vi "AlliGator Save IRFs & Fit Data (Map) HDF5 File v0.6.vi"(0 "File Path":path, 5 "IRFs & Fit Data Map v3":T12 {"Fit Options: Decay Preprocessing Parameters"."# Folds" min=1}, 7 "Decay Fit Options & Parameters v3":T1={"SYNC Period"=0.0, "Fit Options"={"Show Fit Residuals"=FALSE, "Fit Model"=enum."1-Exponential", "Residual Type"=enum."Standard", "Max Decay Percentile"=0.0, "Min Decay Percentile"=0.0, "Show Full Decay"=FALSE, "Weights"=enum."Unweighted", "Fitting Method"=enum."Least Square", "Compute Parameter Uncertainties"=FALSE, "Periodic Boundaries"=FALSE, "Model Calculation"=enum."Simulation", "Period"=0.0, "Termination Criteria"={"Max Iterations"=0, "Max Function Calls"=0, "Max Time"=0.0, "Function Tolerance"=0.0, "Parameter Tolerance"=0.0, "Gradient Tolerance"=0.0, "Min Lambda"=0.0, "Max Lambda"=0.0, "Initial Tick Count"=0}, "Offset Resolution"=0.0, "Use Local IRF"=FALSE, "Fitting Algorithm"=enum."Levenberg-Marquardt", "Show Confidence Interval "=TRUE, "Confidence Level"=95.0}, "Fit Parameter Constraints"=[], "MLE Baseline Offset"=0.0, "MLE Baseline Offset Type"=enum."Absolute"} {"Fit Options"."Confidence Level" min=0.0 max=100.0; "Fit Options"."Offset Resolution" min=0.0; "Fit Options"."Period" min=0.0; "Fit Options"."Min Decay Percentile" min=0.0 max=1.0; "Fit Options"."Max Decay Percentile" min=0.0 max=100.0; "Fit Parameter Constraints"."Max Value" format="%#.3g"; "Fit Parameter Constraints"."Min Value" format="%#.3g"}, 9 "Software + Version":string, 11 "Error In":errorcluster, 12 "[Multiple Decays Fit Parameters SDV]":dbl[][](array[numeric])) -> (4 "File Path out":path, 14 "Time (s)":dbl, 15 "Error Out":errorcluster)   [LabVIEW 2021, in "AlliGator Decay Fit Parameter Map.lvlib"]
doc: "Saves Decay Fit Parameter Map and associated metadata to an HDF5 file."
uses:
  AlliGator Decay Fit Parameter Map.lvlib
  Fits/IRF(X)PSED/Decay Fit Parameters & Derived Quantities List v2.ctl
  Decay Analysis/Decay Preprocessing/AlliGator Decay Preprocessing Parameters.ctl
  Graphs/XY Graph/XY Graph Plot Shift Parameters.ctl
  Graphs/XY Graph/XY Graph Plot Shift Method.ctl
  AlliGator Decay Fit Options & Parameters v3.ctl
  Fits/IRF(X)PSED/Decay Fit Options v3.ctl
  Fits/Decay Convolution/Decay Model.ctl
  Fits/Residual Type.ctl
  Fits/IRF(X)PSED/Fit Weights Type.ctl
  Fits/Non-linear Fitting Method v2.ctl
  Fits/Fit Calculation Method.ctl
  Fits/Non-linear Fitting Algorithm.ctl
  Decay Analysis/Decay Fit/AlliGator Decay Fit Parameter Constraints 2.ctl
  Fits/IRF(X)PSED/Decay Fit Parameters In List.ctl
  Fits/IRF(X)PSED/MLE Baseline Offset Type.ctl
  <vilib>/addons/h5labview2/file/H5Fmode.ctl
  Globals, Variables, Constants/AlliGator Variables List.ctl
  <vilib>/addons/h5labview2/base/lib_path.vi
  <vilib>/addons/h5labview2/base/H5Equery.vi
  <vilib>/addons/h5labview2/dataset/H5Dwrite.llb/H5Dwrite.xnode
  <vilib>/addons/h5labview2/base/hid_t.ctl
  Variant/Variant to Data/Variant to String.vi
  <vilib>/addons/h5labview2/file/H5F.lvlib
  <vilib>/addons/h5labview2/group/H5G.lvlib
  Time/Time.lvlib
  Utilities/Utilities.lvlib
  Strings/Strings.lvlib
  Globals, Variables, Constants/AlliGator Globals, Variables & Constants.lvlib
  Variant/Variant to Data/Variant to Data.lvlib
  Fits/Fits.lvlib
  Graphs/XY Graph/XY Graph Add-Ons.lvlib
  Decay Analysis/Decay Preprocessing/AlliGator Decay Preprocessing.lvlib
  Decay Analysis/Decay Fit/AlliGator Decay Fit.lvlib
  AlliGator IRFs & Fit Data v3.ctl
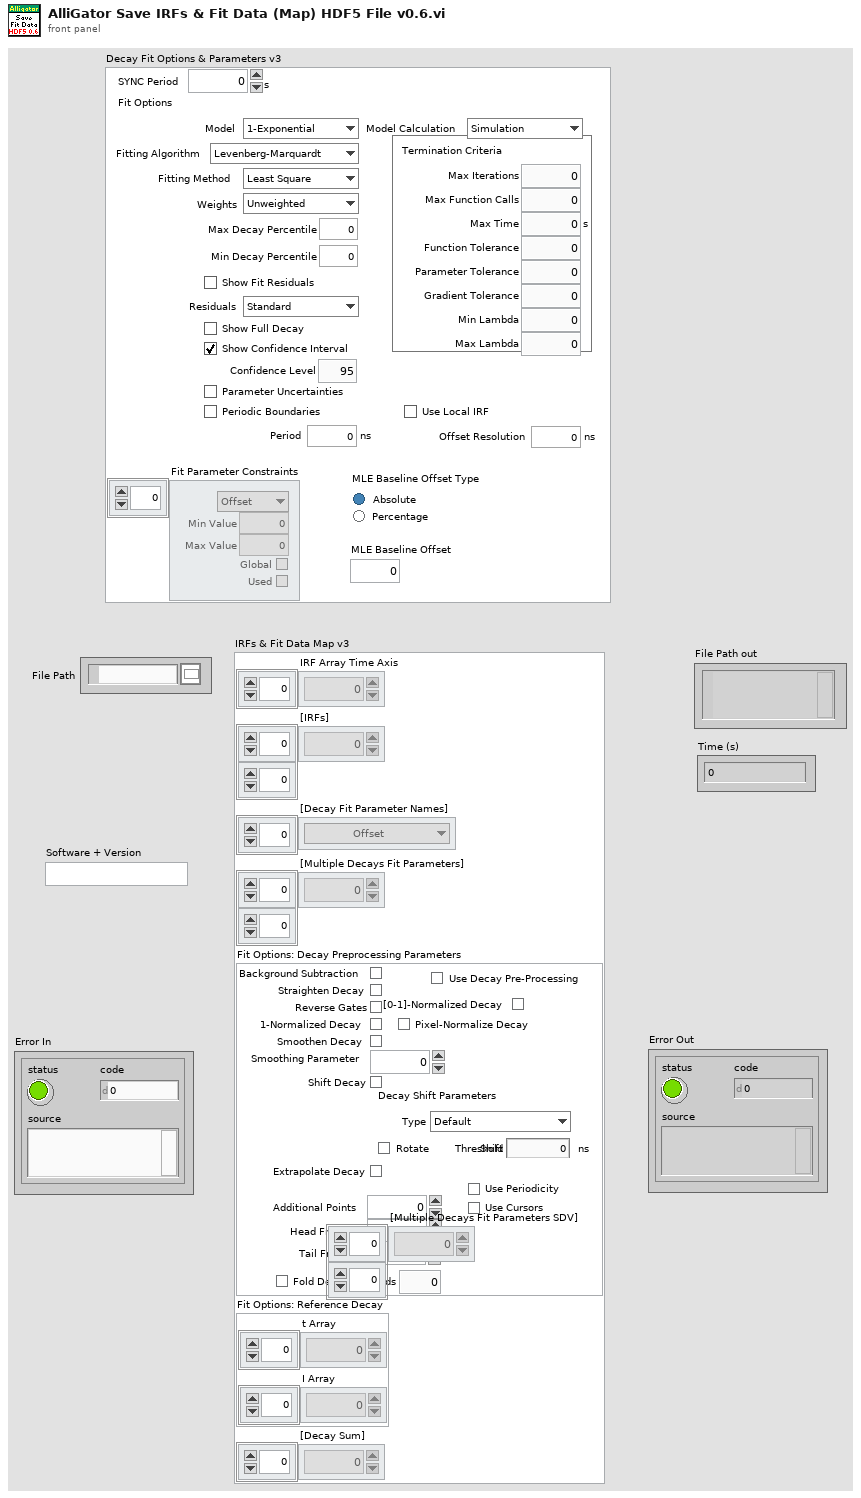
[diagram p1: front panel]
types:
  T1 = typedef "AlliGator Decay Fit Parameter Map.lvlib/AlliGator Decay Fit Options & Parameters v3.ctl" = cluster{"SYNC Period":dbl[unit], "Fit Options":T2, "Fit Parameter Constraints":T9[], "MLE Baseline Offset":dbl, "MLE Baseline Offset Type":T11}
  T2 = typedef "Fits.lvlib/Decay Fit Options v3.ctl" = cluster{"Show Fit Residuals":bool, "Fit Model":T3, "Residual Type":T4, "Max Decay Percentile":dbl, "Min Decay Percentile":dbl, "Show Full Decay":bool, "Weights":T5, "Fitting Method":T6, "Compute Parameter Uncertainties":bool, "Periodic Boundaries":bool, "Model Calculation":T7, "Period":dbl[unit], "Termination Criteria":cluster{"Max Iterations":i32, "Max Function Calls":i32, "Max Time":dbl[unit], "Function Tolerance":dbl, "Parameter Tolerance":dbl, "Gradient Tolerance":dbl, "Min Lambda":dbl, "Max Lambda":dbl, "Initial Tick Count":u32}, "Offset Resolution":dbl[unit], "Use Local IRF":bool, "Fitting Algorithm":T8, "Show Confidence Interval ":bool, "Confidence Level":dbl}
  T3 = typedef "Fits.lvlib/Decay Model.ctl" = enum16{"1-Exponential", "2-Exponentials"}
  T4 = typedef "Fits.lvlib/Residual Type.ctl" = enum16{"Standard", "Normalized", "Reduced"}
  T5 = typedef "Fits.lvlib/Fit Weights Type.ctl" = enum16{"Unweighted", "1/Variance", "Best of All"}
  T6 = typedef "Fits.lvlib/Non-linear Fitting Method v2.ctl" = enum16{"Least Square", "Least Absolute Residual", "Bisquare", "MLE", "-", "Best of All"}
  T7 = typedef "Fits.lvlib/Fit Calculation Method.ctl" = enum16{"Simulation", "Convolution", "Integration"}
  T8 = typedef "Fits.lvlib/Non-linear Fitting Algorithm.ctl" = enum16{"Levenberg-Marquardt", "Trust-Region Dogleg"}
  T9 = typedef "AlliGator Decay Fit.lvlib/AlliGator Decay Fit Parameter Constraints 2.ctl" = cluster{"Fit Parameter":T10, "Min Value":dbl, "Max Value":dbl, "Global":bool, "Used":bool}
  T10 = typedef "Fits.lvlib/Decay Fit Parameters In List.ctl" = enum16{"Offset", "Baseline", "A_1", "tau_1", "A_2", "tau_2"}
  T11 = typedef "Fits.lvlib/MLE Baseline Offset Type.ctl" = enum32{"Absolute", "Percentage"}
  T12 = typedef "AlliGator Decay Fit Parameter Map.lvlib/AlliGator IRFs & Fit Data v3.ctl" = cluster{"IRF Array Time Axis":dbl[], "[IRFs]":dbl[][], "[Decay Fit Parameter Names]":T13[], "[Multiple Decays Fit Parameters]":dbl[][], "Fit Options: Decay Preprocessing Parameters":T14, "Fit Options: Reference Decay":cluster{"t Array":dbl[], "I Array":dbl[]}, "[Decay Sum]":dbl[]}
  T13 = typedef "Fits.lvlib/Decay Fit Parameters & Derived Quantities List v2.ctl" = enum16{"Offset", "Baseline", "A_1", "tau_1", "A_2", "tau_2", "<tau>_a", "f1_a", "f2_a", "<tau>_i", "f1_i", "f2_i", "-", "R^2", "Chi^2"}
  T14 = typedef "AlliGator Decay Preprocessing.lvlib/AlliGator Decay Preprocessing Parameters.ctl" = cluster{"Background Subtraction":bool, "Straighten Decay":bool, "Reverse Gates":bool, "1-Normalized Decay":bool, "Smoothen Decay":bool, "Smoothing Parameter":dbl, "Shift Decay":bool, "Decay Shift Parameters":T15, "Extrapolate Decay":bool, "Additional Points":u32, "Head Fraction":dbl, "Pixel-Normalize Decay":bool, "Use Periodicity":bool, "Use Cursors":bool, "Tail Fraction":dbl, "Use Decay Pre-Processing":bool, "Fold Decay":bool, "# Folds":u32, "[0-1]-Normalized Decay":bool}
  T15 = typedef "XY Graph Add-Ons.lvlib/XY Graph Plot Shift Parameters.ctl" = cluster{"Type":T16, "Shift":dbl[unit], "Threshold":dbl, "Rotate":bool}
  T16 = typedef "XY Graph Add-Ons.lvlib/XY Graph Plot Shift Method.ctl" = enum16{"Default", "CFD", "Threshold", "Cross-Correlation"}
  T17 = typedef "AlliGator Globals, Variables & Constants.lvlib/AlliGator Variables List.ctl" = enum16{"---- GUI ----", "GUI:Initialization Status", "GUI:State Indicators Refnum", "GUI:Original AlliGator Menu Items", "GUI:Current Action Loop State", "GUI:Script in progress", "GUI:Playback", "GUI:Loop Playback", "GUI:Search ROI Used", "GUI:Search ROI", "Decay Graph Max Legend Size", "Intensity Graph Max Legend Size", "Decay Statistics Graph Max Legend Size", "Phasor Graph Max Legend Size", "Phasor Ratio Graph Max Legend Size", "Lifetime Graph Max Legend Size", "---- Files ----", "Files:Export Dataset Frames as Individual Files", "Files:Show Batch Export Help Balloons", "Files:Frames in Dataset", "Files:ptu File Frame Start Indices", "Files:Current Frame in Dataset", "Files:Current Frame Timestamp", "Files:Dataset Loaded", "Files:Dataset Metadata", "Files:Dataset Channel", "Files:Dataset Data Description", "Files:Background Dataset Metadata", "Files:Background Dataset Channel", "Files:Background Dataset Data Description", "Files:Background File Subtraction", "Files:Background File Path", "Files:Background File Pile-up Correction", "Files:Background File Pixel Well Capacity", "Files:Background File Scaling Factor", "Files:Current Dataset Load Settings", "Files:Dataset Path", "Files:ICCD-specific Information", "Files:Macrotime Gate Separation", "------ Python Plugins ------", "Python Plugins:Information", "Python Plugins:Python Session", "Python Plugins:Valid Python Session?", "---- Source Image ----", "Source Image:ROIs", "Source Image:Current ROI", "Source Image:ROI Event Refnum", "X_Source Image:Display Range", "X_Source Image:Palette Information", "X_Source Image:Type of Displayed Image", "X_Time Gate Slider", "Source Image:Palette List", "Source Image:Scale", "Source Image:ROI Overlay Color", "Source Image:Overlay to Erase", "Source Image:Is Displayed Image Accumulated", "Source Image:White Light Image Modified", "Source Image:Mask Image Modified", "---- Image Profile Window ----", "Image Profile:Window Event Refnum", "Image Profile:IntensityType", "Image Profile:Intensity Average Type", "Image Profile:Intensity-weighted SDV", "Image Profile:Box Profile Type", "Image Profile:Window Open", "Image Profile:Plotted Fit Parameter", "------ Phasor Graph -------", "Phasor Graph:Show Line", "---- Phasor Plot ---", "Phasor Plot:Parameters Changed", "Phasor Plot:FLI Dataset Modified since last Calculation", "Phasor Harmonics Data", "Selected Phasor Harmonics", "Phasor Harmonic Manager Event Refnum", "Phasor Plot:ROIs", "Phasor Plot:Current ROI", "Phasor Plot:ROI Event Refnum", "Phasor Plot:Image Reference Points", "Phasor Plot:Computed", "Phasor Plot:Palette Information", "Phasor Plot:Palette List", "Phasor Plot:Phasor Ratio Palette Information", "Phasor Plot:Phasor Ratio Palette List", "Phasor Plot:Image Scale", "Phasor Plot:Image Overlay to Erase", "Phasor Plot:Image Elements to Update", "Phasor Plot:Current Calculation Parameters", "Phasor Plot:Current Calibration Options", "Phasor Plot:Reset Cumulated Phasor Plot", "Phasor Plot:Reference 1", "Phasor Plot:Lifetime Reference 1", "Phasor Plot:Reference 1 Frequency", "Phasor Plot:Reference 2", "Phasor Plot:Lifetime Reference 2", "Phasor Plot:Reference 2 Frequency", "---- Decay Analysis ----", "Number of Selected Decays to Fit", "LS Fit Results", "LAR Fit Results", "BS Fit Results", "Last Decay Max - Min", "Best Fit Parameters", "Best Fit Parameter Names", "Actual Size X", "Actual Size Y", "Binning X", "Binning Y", "Actual # Gates", "Dataset Number", "Gates to...", "Gates Skipped", "Gates to keep", "Gate Step", "Gate Separation", "Reversed Gates", "Pile-up Correction", "Pixel Well Capacity", "Background Subtracted", "Background Subtraction Method", "Background Definition Range", "Background File (deprecated)", "Number of Dataset Accumulated", "Array of Accumulated Dataset Paths", "Do Averaged Datasets", "Destination File Path", "Process Plot Target", "Use 1/D as Phasor Frequency", "---- Decay Fit Parameter Map -----", "Decay Fit Parameter Map:Palette Information", "Decay Fit Parameter Map:Palette List", "Decay Fit Parameter Map:X Resolution", "Decay Fit Parameter Map:Y Resolution", "---- Parameter Map ----", "Parameter Map:Palette Information", "Parameter Map:Palette List", "------- Local Decay Window ---------", "Local Decay Graph Window:Event Refnum", "Local Decay Graph Window:Use normalized IRF for convolution", "----- Miscellaneous ----", "Misc:Skippable Dialog Windows Status"}
  T18 = typedef "H5F.lvlib/H5Fmode.ctl" = enum16{"read-only", "read-write", "overwrite", "create new", "open or create"}
  T19 = typedef "hid_t.ctl" = i64
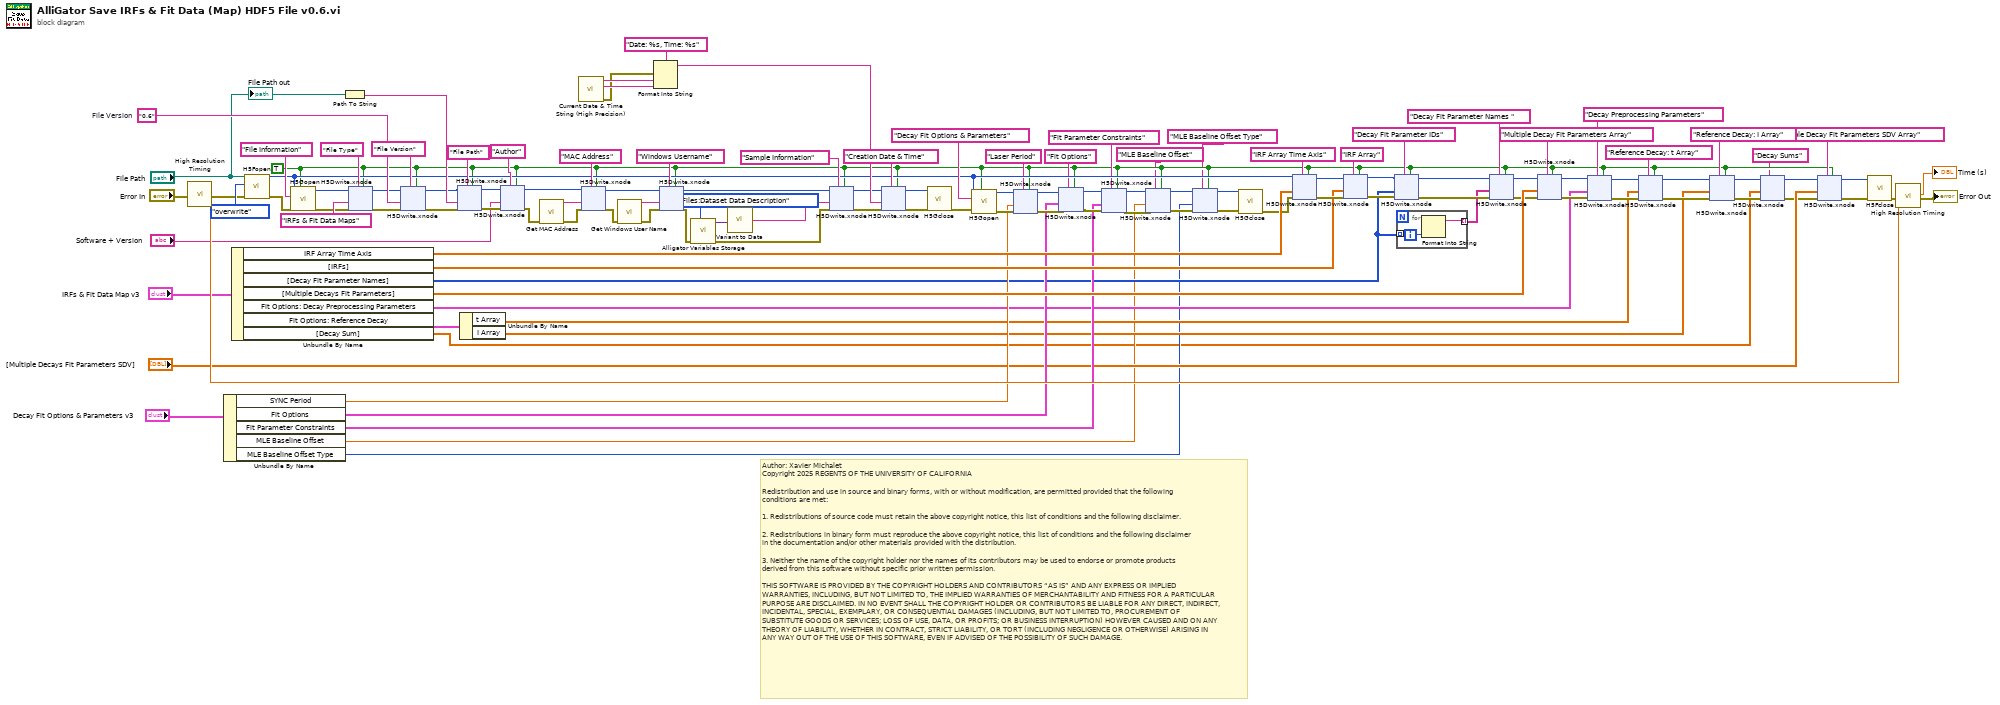
[diagram p0: block diagram]
diagram:
  w114 = "0.6"  # File Version
  w11 = TRUE ("replace? (F)")
  # "Author: Xavier Michalet\nCopyright 2025 REGENTS OF THE UNIVERSITY OF CALIFORNIA\n\nRedistribution and use in source and binary forms, with or without modification, are permitted provided that the following conditions are met:\n\n1. Redistributions of source code must retain the above copyright notice, this list of conditions and the following disclaimer.\n\n2. Redistributions in binary form must reproduce the above copyright notice, this list of conditions and the following disclaimer in the documentation and/or other materials provided with the distribution.\n\n3. Neither the name of the copyright holder nor the names of its contributors may be used to endorse or promote products derived from this software without specific prior written permission.\n\nTHIS SOFTWARE IS PROVIDED BY THE COPYRIGHT HOLDERS AND CONTRIBUTORS “AS IS” AND ANY EXPRESS OR IMPLIED WARRANTIES, INCLUDING, BUT NOT LIMITED TO, THE IMPLIED WARRANTIES OF MERCHANTABILITY AND FITNESS FOR A PARTICULAR PURPOSE ARE DISCLAIMED. IN NO EVENT SHALL THE COPYRIGHT HOLDER OR CONTRIBUTORS BE LIABLE FOR ANY DIRECT, INDIRECT, INCIDENTAL, SPECIAL, EXEMPLARY, OR CONSEQUENTIAL DAMAGES (INCLUDING, BUT NOT LIMITED TO, PROCUREMENT OF SUBSTITUTE GOODS OR SERVICES; LOSS OF USE, DATA, OR PROFITS; OR BUSINESS INTERRUPTION) HOWEVER CAUSED AND ON ANY THEORY OF LIABILITY, WHETHER IN CONTRACT, STRICT LIABILITY, OR TORT (INCLUDING NEGLIGENCE OR OTHERWISE) ARISING IN ANY WAY OUT OF THE USE OF THIS SOFTWARE, EVEN IF ADVISED OF THE POSSIBILITY OF SUCH DAMAGE."
  n1 = call "High Resolution Timing.vi"("Error In"="Error In") -> ("elapsed (relative) seconds"=w117:dbl, "Error Out"=w119:errorcluster)  [unwired: 16 in, 1 out]
  n2 = Unbundle By Name("Decay Fit Options & Parameters v3") -> ("SYNC Period"=w51:dbl[unit], "Fit Options"=w48:T2, "Fit Parameter Constraints"=w47:T9[], "MLE Baseline Offset"=w9:dbl, "MLE Baseline Offset Type"=w8:T11)
  n3 = Unbundle By Name("IRFs & Fit Data Map v3") -> ("IRF Array Time Axis"=w73:dbl[], "[IRFs]"=w72:dbl[][], "[Decay Fit Parameter Names]"=w33:T13[], "[Multiple Decays Fit Parameters]"=w67:dbl[][], "Fit Options: Decay Preprocessing Parameters"=w24:T14, "Fit Options: Reference Decay"=w23:cluster{"t Array":dbl[], "I Array":dbl[]}, "[Decay Sum]"=w1:dbl[])
  n4 = call <vilib>:"H5Fopen.vi"("error in (no error)"=w119, "mode (read-only)"=H5Fmode."overwrite", "path"="File Path") -> ("error out"=w121:errorcluster, "ref out"=w57:T19)  [unwired: 7 in]
  n5 = call <vilib>:"H5Gopen.vi"("create? (F)"=w11, "error in (no error)"=w121, "name"="File Information", "ref in"=w57) -> ("error out"=w109:errorcluster, "group out"=w106:T19)  [unwired: 6 in]
  n6 = Path To String(path="File Path") -> (string=w93:string)
  n7 = xnode "H5Dwrite.xnode"("replace? (F)"=w11, "dataset name"="File Type", "error in (no error)"=w109, "data"="IRFs & Fit Data Maps" ("dataset name"), "ref in"=w106) -> ("error out"=w65:errorcluster, "ref out"=w66:i64)  [unwired: 2 in, 1 out]
  n8 = xnode "H5Dwrite.xnode"("replace? (F)"=w11, "dataset name"="File Version", "error in (no error)"=w65, "data"=w114, "ref in"=w66) -> ("error out"=w64:errorcluster, "ref out"=w63:T19)  [unwired: 2 in, 1 out]
  n9 = xnode "H5Dwrite.xnode"("replace? (F)"=w11, "dataset name"="File Path", "error in (no error)"=w64, "data"=w93, "ref in"=w63) -> ("error out"=w103:errorcluster, "ref out"=w104:T19)  [unwired: 2 in, 1 out]
  n10 = Unbundle By Name(w23) -> ("t Array"=w22:dbl[], "I Array"=w18:dbl[])
  n11 = xnode "H5Dwrite.xnode"("replace? (F)"=w11, "dataset name"="Author", "error in (no error)"=w103, "data"="Software + Version", "ref in"=w104) -> ("error out"=w41:errorcluster, "ref out"=w101:T19)  [unwired: 2 in, 1 out]
  n12 = call "Get MAC Address.vi"("Error In"=w41) -> ("Error Out"=w40:errorcluster, "MAC address"=w98:string)  [unwired: 9 in]
  n13 = call "Current Date & Time String (High Precision).vi"() -> ("Error Out"=w90:errorcluster, "time string"=w91:string, "date string"=w92:string)  [unwired: 8 in, 1 out]
  n14 = xnode "H5Dwrite.xnode"("replace? (F)"=w11, "dataset name"="MAC Address", "error in (no error)"=w40, "data"=w98, "ref in"=w101) -> ("error out"=w39:errorcluster, "ref out"=w100:T19)  [unwired: 2 in, 1 out]
  n15 = call "Get Windows User Name.vi"("Error In"=w39) -> ("Error Out"=w38:errorcluster, "User Name"=w96:string)  [unwired: 9 in]
  n16 = Format Into String(format string="Date: %s, Time: %s", error in=w90, w92, w91) -> (resulting string=w87:string)  [unwired: 1 in, 1 out]
  n17 = xnode "H5Dwrite.xnode"("replace? (F)"=w11, "dataset name"="Windows Username", "error in (no error)"=w38, "data"=w96, "ref in"=w100) -> ("error out"=w79:errorcluster, "ref out"=w85:T19)  [unwired: 2 in, 1 out]
  n18 = call "Alligator Variables Storage.vi"("AlliGator Variable"=AlliGator_Variables_List."Files:Dataset Data Description" ("Alligator Variable"), "Error In"=w79) -> ("Error Out"=w78:errorcluster, "Data out"=w81:variant)  [unwired: 7 in, 1 out]
  n19 = call-poly "Variant to Data.vi"("Variant"=w81) -> ("String"=w80:string)  [unwired: 8 in]
  n20 = xnode "H5Dwrite.xnode"("replace? (F)"=w11, "dataset name"="Sample Information" ("name"), "error in (no error)"=w78, "data"=w80, "ref in"=w85) -> ("error out"=w86:errorcluster, "ref out"=w84:T19)  [unwired: 2 in, 1 out]
  n21 = xnode "H5Dwrite.xnode"("replace? (F)"=w11, "dataset name"="Creation Date & Time", "error in (no error)"=w86, "data"=w87, "ref in"=w84) -> ("error out"=w75:errorcluster, "ref out"=w76:T19)  [unwired: 2 in, 1 out]
  n22 = call <vilib>:"H5Gclose.vi"("error in (no error)"=w75, "group in"=w76) -> ("error out"=w62:errorcluster)  [unwired: 9 in]
  n23 = call <vilib>:"H5Gopen.vi"("create? (F)"=w11, "error in (no error)"=w62, "name"="Decay Fit Options & Parameters" ("dataset name"), "ref in"=w57) -> ("error out"=w60:errorcluster, "group out"=w59:T19)  [unwired: 6 in]
  n24 = xnode "H5Dwrite.xnode"("replace? (F)"=w11, "dataset name"="Laser Period", "error in (no error)"=w60, "data"=w51, "ref in"=w59) -> ("error out"=w56:errorcluster, "ref out"=w54:T19)  [unwired: 2 in, 1 out]
  n25 = xnode "H5Dwrite.xnode"("replace? (F)"=w11, "dataset name"="Fit Options", "error in (no error)"=w56, "data"=w48, "ref in"=w54) -> ("error out"=w55:errorcluster, "ref out"=w53:i64)  [unwired: 2 in, 1 out]
  n26 = xnode "H5Dwrite.xnode"("replace? (F)"=w11, "dataset name"="Fit Parameter Constraints", "error in (no error)"=w55, "data"=w47, "ref in"=w53) -> ("error out"=w17:errorcluster, "ref out"=w16:i64)  [unwired: 2 in, 1 out]
  n27 = xnode "H5Dwrite.xnode"("replace? (F)"=w11, "dataset name"="MLE Baseline Offset", "error in (no error)"=w17, "data"=w9, "ref in"=w16) -> ("error out"=w15:errorcluster, "ref out"=w13:i64)  [unwired: 2 in, 1 out]
  n28 = xnode "H5Dwrite.xnode"("replace? (F)"=w11, "dataset name"="MLE Baseline Offset Type", "error in (no error)"=w15, "data"=w8, "ref in"=w13) -> ("error out"=w14:errorcluster, "ref out"=w12:i64)  [unwired: 2 in, 1 out]
  n29 = call <vilib>:"H5Gclose.vi"("error in (no error)"=w14, "group in"=w12) -> ("error out"=w58:errorcluster)  [unwired: 9 in]
  n30 = xnode "H5Dwrite.xnode"("replace? (F)"=w11, "dataset name"="IRF Array Time Axis", "error in (no error)"=w58, "data"=w73, "ref in"=w57) -> ("error out"=w112:errorcluster, "ref out"=w113:T19)  [unwired: 2 in, 1 out]
  n31 = xnode "H5Dwrite.xnode"("replace? (F)"=w11, "dataset name"="IRF Array", "error in (no error)"=w112, "data"=w72, "ref in"=w113) -> ("error out"=w70:errorcluster, "ref out"=w71:T19)  [unwired: 2 in, 1 out]
  n32 = xnode "H5Dwrite.xnode"("replace? (F)"=w11, "dataset name"="Decay Fit Parameter IDs" ("name"), "error in (no error)"=w70, "data"=w33, "ref in"=w71) -> ("error out"=w36:errorcluster, "ref out"=w37:i64)  [unwired: 2 in, 1 out]
  n33 = for {
    tunnel: w33 -> [w125] mode=indexing
    tunnel: [w124] -> w32 mode=indexing
    n34 = Format Into String(w125) -> (resulting string=w124:string)  [unwired: 3 in, 1 out]
  }
  n35 = xnode "H5Dwrite.xnode"("replace? (F)"=w11, "dataset name"="Decay Fit Parameter Names " ("name"), "error in (no error)"=w36, "data"=w32, "ref in"=w37) -> ("error out"=w35:errorcluster, "ref out"=w34:T19)  [unwired: 2 in, 1 out]
  n36 = xnode "H5Dwrite.xnode"("replace? (F)"=w11, "dataset name"="Multiple Decay Fit Parameters Array" ("name"), "error in (no error)"=w35, "data"=w67, "ref in"=w34) -> ("error out"=w28:errorcluster, "ref out"=w30:T19)  [unwired: 2 in, 1 out]
  n37 = xnode "H5Dwrite.xnode"("replace? (F)"=w11, "dataset name"="Decay Preprocessing Parameters" ("name"), "error in (no error)"=w28, "data"=w24, "ref in"=w30) -> ("error out"=w27:errorcluster, "ref out"=w29:i64)  [unwired: 2 in, 1 out]
  n38 = xnode "H5Dwrite.xnode"("replace? (F)"=w11, "dataset name"="Reference Decay: t Array" ("name"), "error in (no error)"=w27, "data"=w22, "ref in"=w29) -> ("error out"=w21:errorcluster, "ref out"=w20:T19)  [unwired: 2 in, 1 out]
  n39 = xnode "H5Dwrite.xnode"("replace? (F)"=w11, "dataset name"="Reference Decay: I Array" ("name"), "error in (no error)"=w21, "data"=w18, "ref in"=w20) -> ("error out"=w5:errorcluster, "ref out"=w6:T19)  [unwired: 2 in, 1 out]
  n40 = xnode "H5Dwrite.xnode"("dataset name"="Decay Sums" ("name"), "error in (no error)"=w5, "data"=w1, "ref in"=w6) -> ("error out"=w3:errorcluster, "ref out"=w4:i64)  [unwired: 3 in, 1 out]
  n41 = xnode "H5Dwrite.xnode"("replace? (F)"=w11, "dataset name"="Multiple Decay Fit Parameters SDV Array" ("name"), "error in (no error)"=w3, "data"="[Multiple Decays Fit Parameters SDV]", "ref in"=w4) -> ("error out"=w44:errorcluster, "ref out"=w45:T19)  [unwired: 2 in, 1 out]
  n42 = call <vilib>:"H5Fclose.vi"("error in (no error)"=w44, "ref"=w45) -> ("error out"=w123:errorcluster)  [unwired: 9 in]
  n43 = call "High Resolution Timing.vi"("relative seconds (NaN)"=w117, "Error In"=w123) -> ("elapsed (relative) seconds"=→"Time (s)":dbl, "Error Out"=→"Error Out":errorcluster)  [unwired: 15 in, 1 out]
  "File Path out" <- "File Path"
